vi "G#Object_CleanUp.vi"(1 "full class name (\"\")":string, 5 "error in (no error)":errorcluster) -> (15 "any dead objects?":bool, 19 "error out":errorcluster)   [LabVIEW 2020, in "G#Object.lvclass"]
doc: "Cleans up the specified class and remove all \"dead\" object. \"Dead\" object could occur if LabVIEW garbage collector removes objects because the object creating top-level VI stops executing."
uses:
  G#Object.lvclass
  G#Object.lvclass/G#Object.ctl
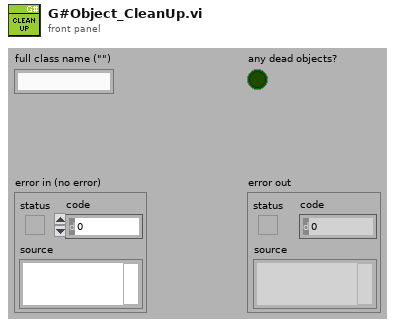
[diagram p1: front panel]
types:
  T1 = cluster{"full class name (\"\")":string, "Ref":refnum<class "G#Object.lvclass">}
  T2 = cluster{"full class name (\"\")":string, "Ref":refnum<class "G#Object.lvclass">}[]
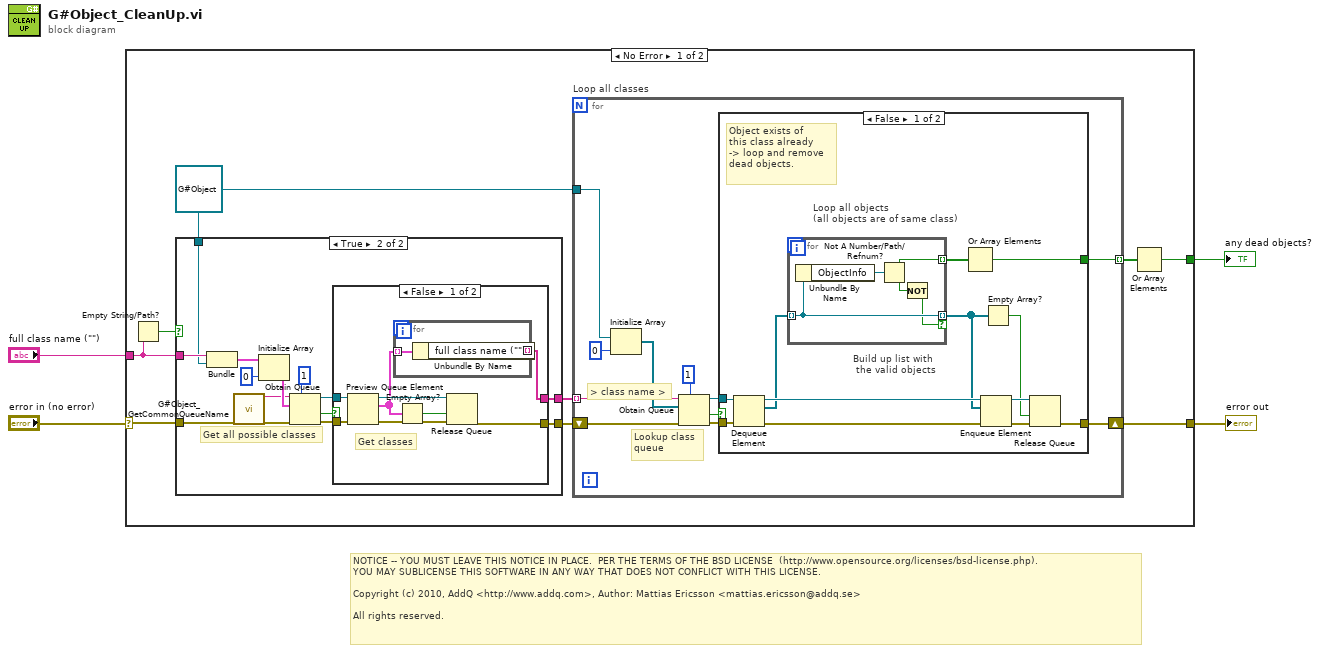
[diagram p0: block diagram]
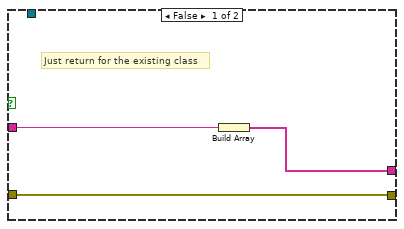
[diagram p2: hidden frame]
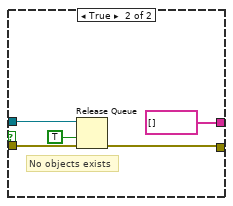
[diagram p3: hidden frame]
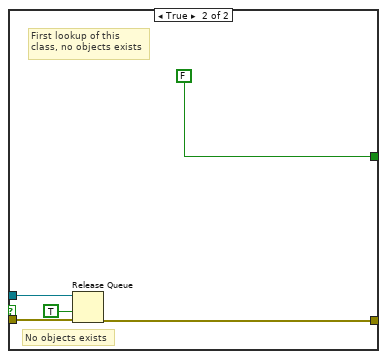
[diagram p4: hidden frame]
diagram:
  # "NOTICE -- YOU MUST LEAVE THIS NOTICE IN PLACE.  PER THE TERMS OF THE BSD LICENSE  (http://www.opensource.org/licenses/bsd-license.php).\nYOU MAY SUBLICENSE THIS SOFTWARE IN ANY WAY THAT DOES NOT CONFLICT WITH THIS LICENSE.\n\nCopyright (c) 2010, AddQ <http://www.addq.com>, Author: Mattias Ericsson <mattias.ericsson@addq.se>\n\nAll rights reserved."
  n1 = case shown="No Error" "error in (no error)" {
    selector: "error in (no error)" -> [w11 w78]
    tunnel: [w10 w78] -> w3
    tunnel: "full class name (\"\")" -> [w8 _]
    tunnel: [w5 _] -> w1
    frame No Error {
      w7 = refnum<class "G#Object.lvclass"> refnum ("Ref")
      n2 = Empty String/Path?(string/path=w8) -> (empty?=w9:bool)
      n3 = case shown="True" w9 {
        tunnel: [w15 w24] -> w13
        tunnel: [w16 w23] -> w12
        tunnel: w11 -> [w16 w19]
        tunnel: w8 -> [w14 w21]
        tunnel: w7 -> [_ w20]
        frame False {
          # "Just return for the existing class"
          n4 = Build Array(w14) -> (w15:string[])
        }
        frame True {
          # "Get all possible classes"
          n5 = Bundle("full class name (\"\")"=w21, "Ref"=w20) -> (w22:T1)  [unwired: 1 in]
          n6 = call "G#Object_GetCommonQueueName.vi"("error in (no error)"=w19) -> ("queue name"=w17:string, "error out"=w18:errorcluster)  [unwired: 17 in]
          n7 = Initialize Array(w22, 0 ("dimension size")) -> (w25:T2)
          n8 = Obtain Queue(max queue size (-1, unlimited)=1, name (unnamed)=w17, element data type=w25, error in (no error)=w18) -> (queue out=w28:refnum<queue>, created new?=w30:bool, error out=w29:errorcluster)  [unwired: 1 in]
          n9 = case shown="False" w30 {
            tunnel: w29 -> [w38 w42]
            tunnel: w28 -> [w37 w43]
            tunnel: [w33 string[] []] -> w24
            tunnel: [w36 w45] -> w23
            frame False {
              # "Get classes"
              n10 = Preview Queue Element(queue=w37, error in (no error)=w38) -> (queue out=w34:refnum<queue>, element=w32:T2, error out=w35:errorcluster)  [unwired: 1 in, 1 out]
              n11 = for {
                tunnel: [w40] -> w33 mode=indexing
                tunnel: w32 -> [w39] mode=indexing
                n12 = Unbundle By Name(w39) -> ("full class name (\"\")"=w40:string)
              }
              n13 = Empty Array?(array=w32) -> (empty?=w31:bool)
              n14 = Release Queue(queue=w34, force destroy? (F)=w31, error in (no error)=w35) -> (error out=w36:errorcluster)  [unwired: 2 out]
            }
            frame True {
              # "No objects exists"
              n15 = Release Queue(queue=w43, force destroy? (F)=TRUE, error in (no error)=w42) -> (error out=w45:errorcluster)  [unwired: 2 out]
            }
          }
        }
      }
      n16 = for "Loop all classes" {
        shift-right: [w47] -> w10
        shift-left: w12 -> [w52]
        tunnel: w13 -> [w51] mode=indexing
        tunnel: w7 -> [w48]
        tunnel: [w46] -> w6 mode=indexing
        # "> class name >"
        # "Lookup class\nqueue"
        n17 = Initialize Array(w48, 0 ("dimension size")) -> (w50:refnum<class "G#Object.lvclass">[])
        n18 = Obtain Queue(max queue size (-1, unlimited)=1, name (unnamed)=w51, element data type=w50, error in (no error)=w52) -> (queue out=w53:refnum<queue>, created new?=w54:bool, error out=w55:errorcluster)  [unwired: 1 in]
        n19 = case shown="False" w54 {
          tunnel: w55 -> [w67 w74]
          tunnel: w53 -> [w66 w75]
          tunnel: [w68 w73] -> w47
          tunnel: [w61 FALSE] -> w46
          frame False {
            # "Build up list with\n the valid objects"
            # "Loop all objects\n(all objects are of same class)"
            # "Object exists of\nthis class already\n-> loop and remove\ndead objects."
            n20 = Dequeue Element(queue=w66, error in (no error)=w67) -> (queue out=w64:refnum<queue>, element=w57:refnum<class "G#Object.lvclass">[], error out=w65:errorcluster)  [unwired: 1 in, 1 out]
            n21 = for {
              tunnel: w57 -> [w71] mode=indexing
              tunnel: [w70] -> w60 mode=indexing
              tunnel: [w71] -> w59 mode=indexing if=w69
              n22 = Unbundle By Name(w71) -> ("ObjectInfo"=w72:refnum<queue>)
              n23 = Not A Number/Path/Refnum?(number/path/refnum=w72) -> (NaN/Path/Refnum?=w70:bool)
              n24 = Not(x=w70) -> (.not. x?=w69:bool)
            }
            n25 = Or Array Elements(Boolean array=w60) -> (logical OR=w61:bool)
            n26 = Enqueue Element(queue=w64, element=w59, error in (no error)=w65) -> (queue out=w62:refnum<queue>, error out=w63:errorcluster)  [unwired: 1 in, 1 out]
            n27 = Empty Array?(array=w59) -> (empty?=w58:bool)
            n28 = Release Queue(queue=w62, force destroy? (F)=w58, error in (no error)=w63) -> (error out=w68:errorcluster)  [unwired: 2 out]
          }
          frame True {
            # "No objects exists"
            # "First lookup of this\nclass, no objects exists"
            n29 = Release Queue(queue=w75, force destroy? (F)=TRUE, error in (no error)=w74) -> (error out=w73:errorcluster)  [unwired: 2 out]
          }
        }
      }
      n30 = Or Array Elements(Boolean array=w6) -> (logical OR=w5:bool)
    }
    frame Error {
    }
  }
  "error out" <- w3
  "any dead objects?" <- w1
